vi "OFBS_decodeParameters.vi"(1 "Parameters":i32[](array[numeric]), 2 "Trial":dbl[][](array[numeric])) -> (0 "FeatureVector":dbl[](array[numeric]))   [LabVIEW 2016, in "Optimal Frequency Bands Search.lvlib"]
doc: "Функция выполняет декодирование параметров (фенотипа)"
uses:
  Optimal Frequency Bands Search.lvlib
panel:
  # "This VI is a part of BCI Design library, http://www.ru-bci.org \nCopyright © 2020, Sotnikov Peter, All rights reserved. License: GNU GPLv3"
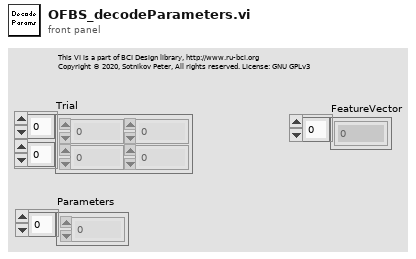
[diagram p1: front panel]
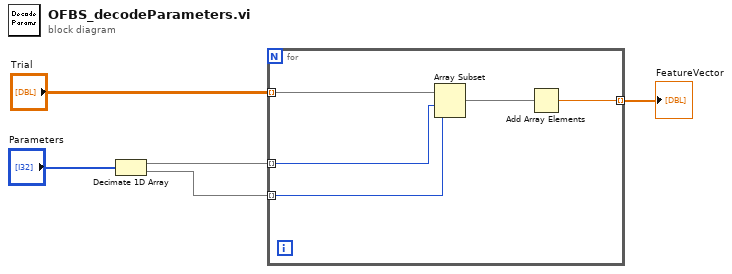
[diagram p0: block diagram]
diagram:
  n1 = Decimate 1D Array "Decimate 1D Array"("Parameters") -> (w2:i32[], w1:i32[])
  n2 = for {
    tunnel: "Trial" -> [w10] mode=indexing
    tunnel: [w6] -> w4 mode=indexing
    tunnel: w2 -> [w9] mode=indexing
    tunnel: w1 -> [w8] mode=indexing
    n3 = Array Subset "Array Subset"(array=w10, index=w9, length=w8) -> (w7:dbl[])
    n4 = Add Array Elements(numeric array=w7) -> (sum=w6:dbl)
  }
  "FeatureVector" <- w4
